vi "cRIO_EPTx_FPGA_MulInj2.vi"() -> ()   [LabVIEW 2020]
uses:
  <vilib>/Platform/TimedLoop/XDataNode/XDataNode.xnode
  <vilib>/Platform/TimedLoop/XDataNode/nitl_modes.ctl
  <vilib>/Platform/TimedLoop/XDataNode/XDNodeRunTimeDep.lvlib
  <vilib>/Platform/TimedLoop/XDataNode/wakeup.ctl
  <vilib>/Platform/TimedLoop/XDataNode/timing_clust.ctl
  <vilib>/Powertrain Controls/Device Drivers/Engine Position Tracking/EPTx/RevA/FPGA/EPTx - RevA - FPGA.lvlib
  <vilib>/Powertrain Controls/Device Drivers/Engine Position Tracking/EPTx/RevA/FPGA/Extras/Command Sequence - 8e.vi
  <vilib>/eio/EIONode/EIONode.xnode
  <vilib>/rvi/eio/common/nirviEmuTemplateMethod_errors.vi
panel:
  in  "GlobalTrigger":bool
  in  "SeqReset":bool
  out "Cmd":bool
  out "Paused":bool
  out "CmdTimer":u32
  out "SeqPointer":u8
  in  "ContinueSeq8":bool
  in  "ContinueSeq7":bool
  in  "ContinueSeq6":bool
  in  "ContinueSeq5":bool
  in  "ContinueSeq4":bool
  in  "ContinueSeq3":bool
  in  "ContinueSeq2":bool
  in  "ContinueSeq1":bool
  in  "CmdLevelSeq8":bool
  in  "CmdLevelSeq7":bool
  in  "CmdLevelSeq6":bool
  in  "CmdLevelSeq5":bool
  in  "CmdLevelSeq4":bool
  in  "CmdLevelSeq3":bool
  in  "CmdLevelSeq2":bool
  in  "CmdLevelSeq1":bool
  in  "DurationSeq8":u32
  in  "DurationSeq7":u32
  in  "DurationSeq6":u32
  in  "DurationSeq5":u32
  in  "DurationSeq4":u32
  in  "DurationSeq3":u32
  in  "DurationSeq2":u32
  in  "DurationSeq1":u32
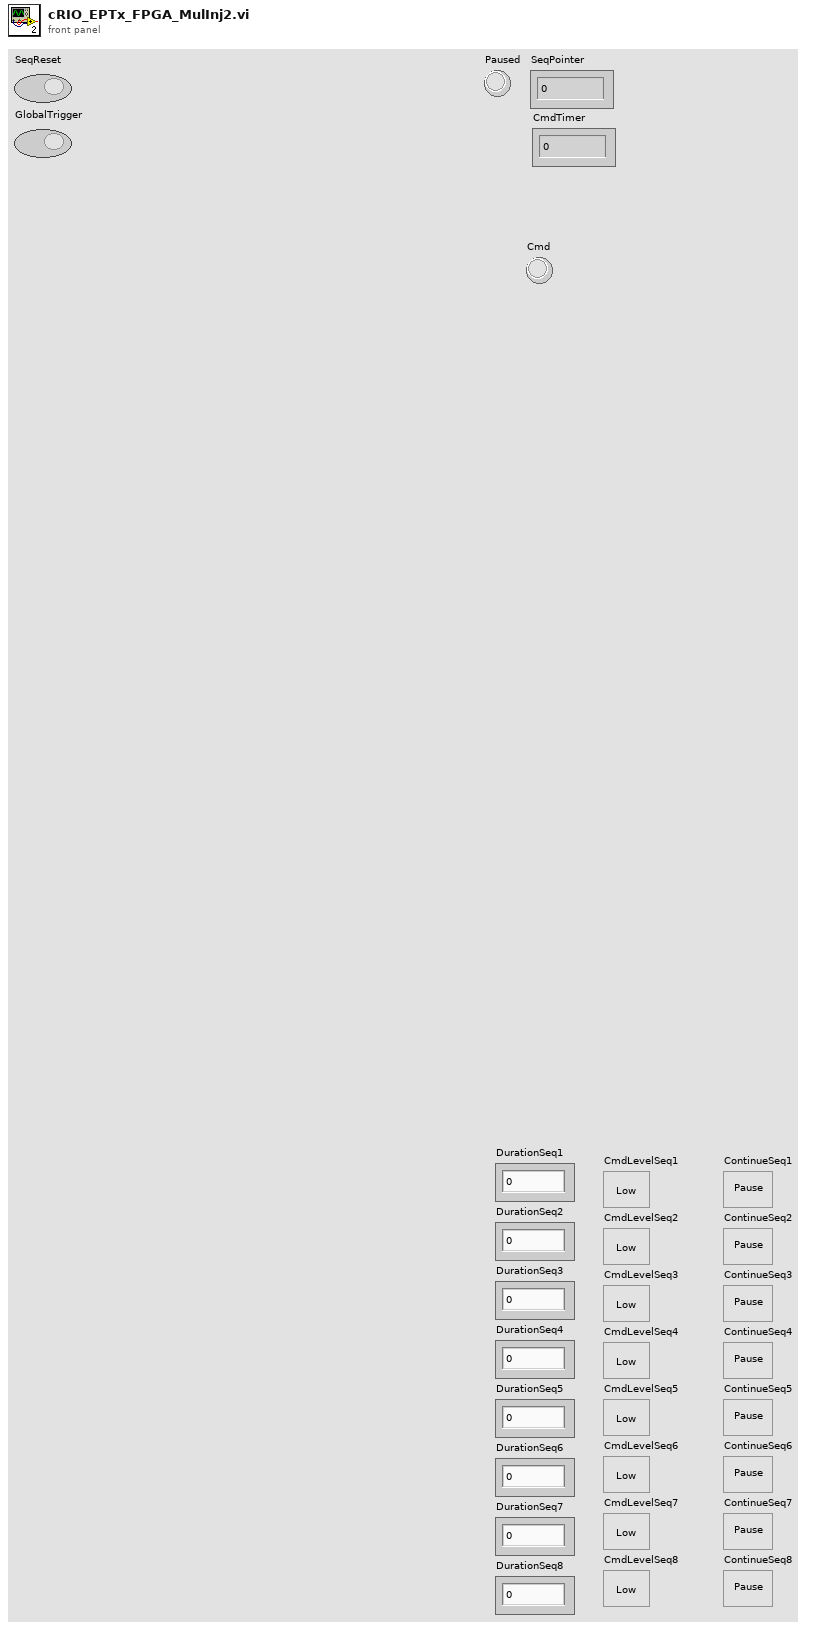
[diagram p1: front panel]
types:
  T1 = typedef "XDNodeRunTimeDep.lvlib/timing_clust.ctl" = cluster{"Expected End [f-1]":u64, "Actual End [f-1]":u64, "Finished Late? [f-1]":bool, "Expected End [i-1]":u64, "Actual End [i-1]":u64, "Finished Late? [i-1]":bool, "Expected Start [i]":u64, "Actual Start [i]":u64, "Expected Start [f]":u64, "Actual Start [f]":u64, "Source Name":string, "Structure Name":string, "Period":i64, "Deadline":i64, "Offset":i64, "Start":i64, "Priority":i32, "Timeout":i32, "Mode":T2, "Wakeup Reason":T3, "Error":errorcluster, "Source Type":string, "Secondary Source Type":string, "Global End Time":u64, "Global Start Time":u64, "Frame Duration":u64, "Iteration Duration":u64, "Assigned CPU":i32, "I/O Scan Engine Mode":u32}
  T2 = typedef "XDNodeRunTimeDep.lvlib/nitl_modes.ctl" = enum32{"No Change", "Process missed periods, maintain original phase", "Discard missed periods, maintain original phase", "Process missed periods, ignore original phase", "Discard missed periods, ignore original phase"}
  T3 = typedef "XDNodeRunTimeDep.lvlib/wakeup.ctl" = enum32{"Normal", "Aborted", "Asynchronous wakeup", "Timing source error", "Timed loop error", "Timeout"}
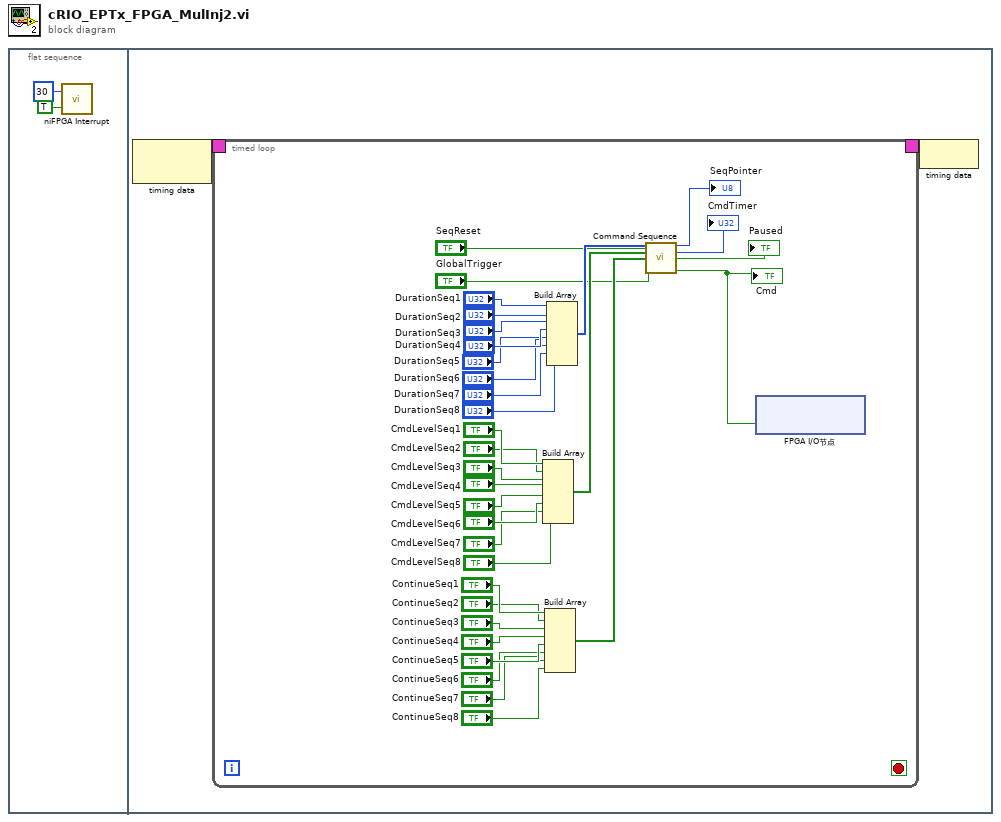
[diagram p0: block diagram]
diagram:
  n1 = flat-sequence {
    frame #0 {
      n2 = call <vilib>:"niFPGA Interrupt.vi"("Wait Until Cleared (F)"=TRUE, "IRQ Number (0)"=u8 30) -> ()  [unwired: 1 in]
    }
    frame #1 {
      n3 = node-c288() -> (w4:T1)  [unwired: 1 in]
      n4 = timed-loop {
        timing: w4 -> [_]
        timing-out: [_] -> w3
        stop <- _ stop-if-true
        n5 = Build Array("CmdLevelSeq1", "CmdLevelSeq2", "CmdLevelSeq3", "CmdLevelSeq4", "CmdLevelSeq5", "CmdLevelSeq6", "CmdLevelSeq7", "CmdLevelSeq8") -> (w12:bool[])
        n6 = Build Array("ContinueSeq1", "ContinueSeq2", "ContinueSeq3", "ContinueSeq4", "ContinueSeq5", "ContinueSeq6", "ContinueSeq7", "ContinueSeq8") -> (w11:bool[])
        n7 = Build Array("DurationSeq1", "DurationSeq2", "DurationSeq3", "DurationSeq4", "DurationSeq5", "DurationSeq6", "DurationSeq7", "DurationSeq8") -> (w29:u32[])
        n8 = call-poly <vilib>:"Command Sequence.vi"("DurationSeq"=w29, "CmdLevelSeq"=w12, "ContinueSeq"=w11, "SeqReset"="SeqReset", "GlobalTrigger"="GlobalTrigger") -> ("SeqPointer"=→"SeqPointer":u8, "CmdTimer"=→"CmdTimer":u32, "Paused"=→"Paused":bool, "Cmd"=w5:bool)  [unwired: 7 in]
        "Cmd" <- w5
        n9 = xnode "FPGA I/O节点"("模块6/DIO5"=w5) -> ()  [unwired: 1 in, 1 out]
      }
      n10 = node-c288(w3) -> ()
    }
  }
